vi "var_OCTzHomeDir.vi"() -> ()   [LabVIEW 2016]
panel:
  in  "OCTz Home Dir":bool
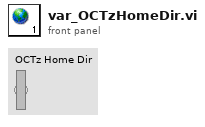
[diagram p1: front panel]
diagram:
